vi "Configure Channel Probe.vi"(4 "Probe Model Number (0: P5205)":i32(ring) items=["P5205", "P5210", "P6205", "P6241", "P6243", "P6245", "P6246", "P6247", "P6248", "P6249", "P6250", "P6251", "P670X", "P671X", "TCP202"], 5 "Set Probe Model Number (F: Disable)":bool, 6 "Probe Signal Type (1: Single-ended)":i32(ring)=1 items=["Differential", "Single-ended"], 7 "Skew Factor (1E-7 S)":dbl=1e-07, 8 "error in (no error)":errorcluster, 9 "Probe Head Type (8: NONE)":i32(ring)=8 items=["Single- ended, 0dB", "Single- ended, 6dB", "Single- ended, 12dB", "Single- ended, 20dB", "Differential, 0dB", "Differential, 6dB", "Differential, 12dB", "Differential, 20dB", "NONE"], 10 "Channel Name (0: Channel 1)":i32(ring) items=["Channel 1", "Channel 2", "Channel 3", "Channel 4"], 11 "VISA resource name":refnum<visa-resource-name>) -> (0 "error out":errorcluster, 3 "VISA resource name out":refnum<visa-resource-name>)   [LabVIEW 2015, in "Agilent 2000 3000 X-Series.lvlib"]
doc: "Configures the channel probe."
uses:
  <instrlib>/Agilent 2000 3000 X-Series/Agilent 2000 3000 X-Series.lvlib
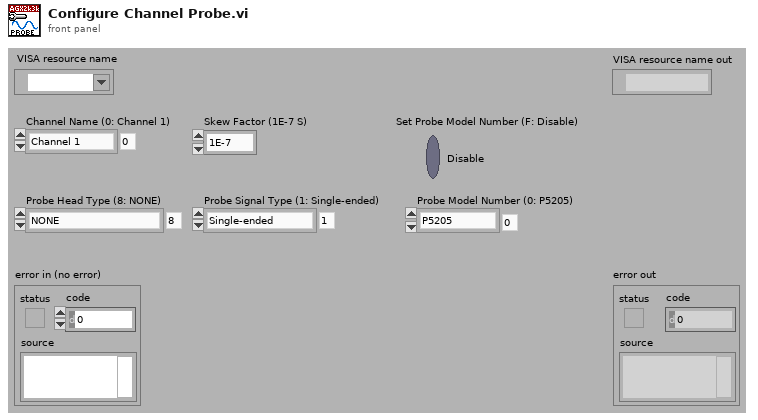
[diagram p1: front panel]
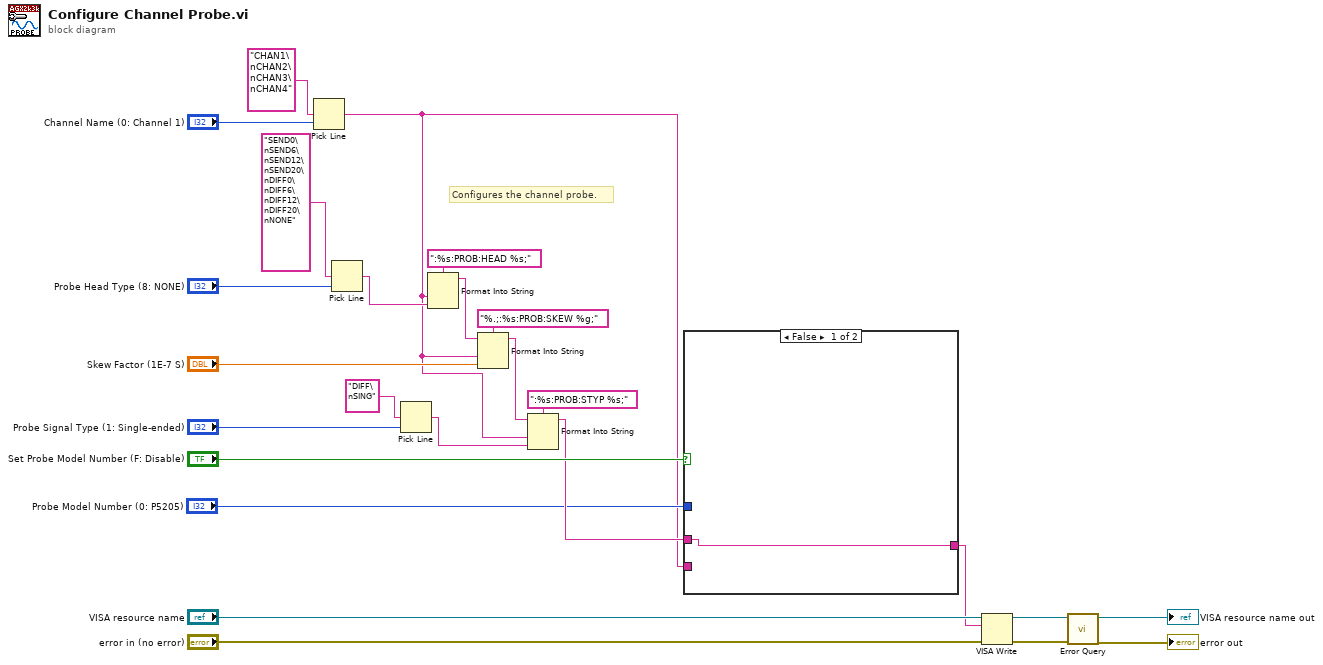
[diagram p0: block diagram]
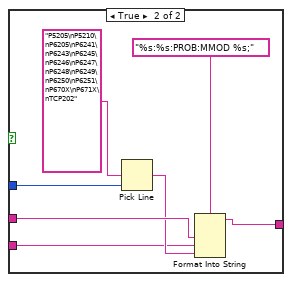
[diagram p2: hidden frame]
diagram:
  # "Configures the channel probe."
  n1 = Pick Line(multi-line string="CHAN1\nCHAN2\nCHAN3\nCHAN4", line index="Channel Name (0: Channel 1)") -> (output string=w1:string)  [unwired: 1 out]
  n2 = Pick Line(multi-line string="SEND0\nSEND6\nSEND12\nSEND20\nDIFF0\nDIFF6\nDIFF12\nDIFF20\nNONE", line index="Probe Head Type (8: NONE)") -> (output string=w22:string)  [unwired: 1 out]
  n3 = Pick Line(multi-line string="DIFF\nSING", line index="Probe Signal Type (1: Single-ended)") -> (output string=w14:string)  [unwired: 1 out]
  n4 = Format Into String(format string=":%s:PROB:HEAD %s;", w1, w22) -> (resulting string=w21:string)  [unwired: 2 in, 1 out]
  n5 = Format Into String(format string="%.;:%s:PROB:SKEW %g;", initial string=w21, w1, "Skew Factor (1E-7 S)") -> (resulting string=w16:string)  [unwired: 1 in, 1 out]
  n6 = Format Into String(format string=":%s:PROB:STYP %s;", initial string=w16, w1, w14) -> (resulting string=w5:string)  [unwired: 1 in, 1 out]
  n7 = case shown="False" "Set Probe Model Number (F: Disable)" {
    tunnel: w5 -> [w26 w31]
    tunnel: [w26 w29] -> w4
    tunnel: "Probe Model Number (0: P5205)" -> [_ w33]
    tunnel: w1 -> [_ w28]
    frame False {
    }
    frame True {
      n8 = Pick Line(multi-line string="P5205\nP5210\nP6205\nP6241\nP6243\nP6245\nP6246\nP6247\nP6248\nP6249\nP6250\nP6251\nP670X\nP671X\nTCP202", line index=w33) -> (output string=w30:string)  [unwired: 1 in]
      n9 = Format Into String(format string="%s:%s:PROB:MMOD %s;", w31, w28, w30) -> (resulting string=w29:string)  [unwired: 2 in, 1 out]
    }
  }
  n10 = VISA Write(VISA resource name="VISA resource name", write buffer=w4, error in (no error)="error in (no error)") -> (VISA resource name out=w11:refnum<visa-resource-name>, error out=w10:errorcluster)  [unwired: 1 out]
  n11 = call <instrlib>:"Error Query.vi"("error in (no error)"=w10, "VISA resource name"=w11) -> ("error out"=→"error out":errorcluster, "VISA resource name out"=→"VISA resource name out":refnum<visa-resource-name>)  [unwired: 8 out]
